vi "AlGaInPAs_run_dil_v11.vi"(2 "Debug Mode":bool, 3 "Elapsed Time(s)":dbl, 4 "State":enum16{"Edit", "Start", "Run", "End", "Idle"}(ring), 5 "Argument List In":string[](array[string])) -> (0 "Status Out":string, 1 "Argument List Out":string[](array[string]))   [LabVIEW 2011]
panel:
  out "Prep-Ga var":bool
  out "run started":bool
  out "first":bool=TRUE
  out "total time":dbl
  out "is OK?":bool
  out "AsH3?":bool
  out "PH3?":bool
  out "In?":bool
  out "Ga?":bool
  out "Al?":bool
  in  "Run As":bool caption="Run"
  in  "AsH3 Flow":dbl caption="AsH3 Flow (0-10 sccm)" format="%.2f"
  in  "P Flow":dbl caption="P Flow (0-100 sccm)" format="%.2f"
  in  "Run P":bool caption="Run"
  in  "In Flow":dbl caption="In Flow (0-100 sscm)" format="%.2f"
  in  "Run In":bool caption="Run"
  in  "Run Al":bool caption="Run"
  in  "Al Flow":dbl caption="Al Flow (0-100 sscm)" format="%.2f"
  in  "Cancel":bool
  in  "OK":bool
  out "tTotal(s) 2":dbl
  in  "Ga Tab Control":enum32{"Page 1", "Page 2"}(tab)
  in  "Ga Dilution":bool caption="Dilute"
  in  "Ga Flow":dbl caption="Ga Flow (0-10 sscm)" format="%.2f"
  in  "Run Ga":bool caption="Run"
  in  "GAMFC1":dbl=1.0 caption="R1 (0-10 sscm)" format="%.2f"
  out "GAMFC2 set":dbl caption="R2 (0-100 sscm)" format="%.2f"
  in  "GAMFC3":dbl=100.0 caption="R3 (0-1000 sscm)" format="%.1f"
  out "GAMFC1 set":dbl caption="R1 (0-10 sscm)" format="%.2f"
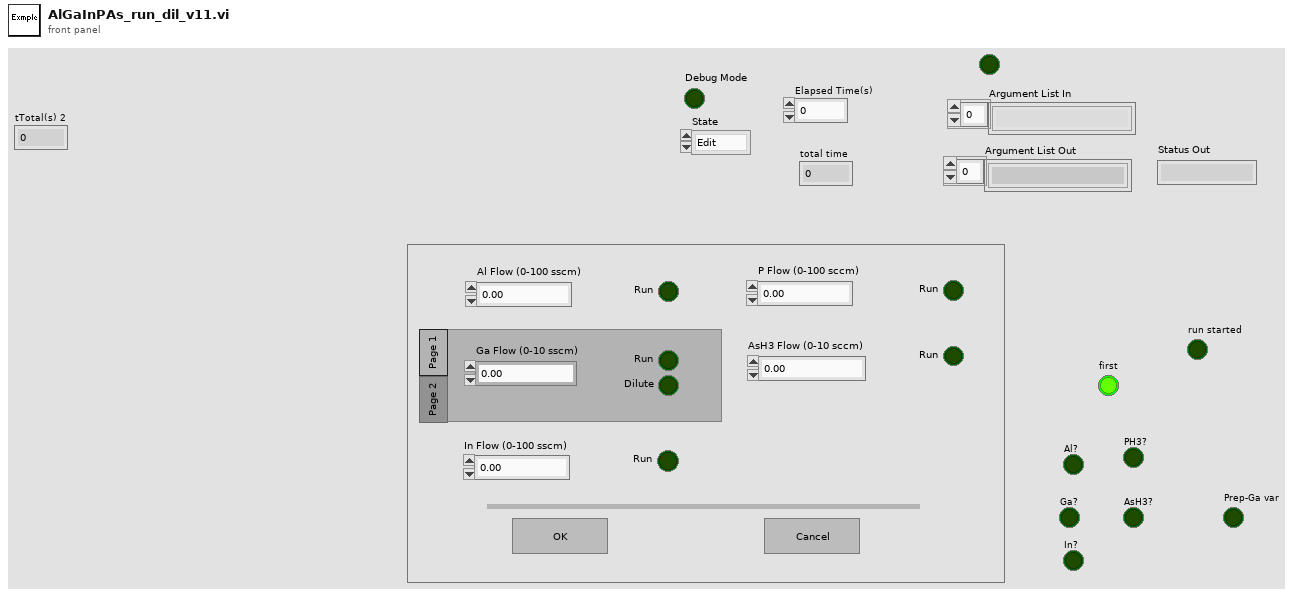
[diagram p1: front panel]
types:
  T1 = enum16{"Discrete", "Continuous", "Instantaneous", "Finite"}
  T2 = enum32{"Invalid", "Default", "Floating", "Floating/Auto-Hide", "Modal"}
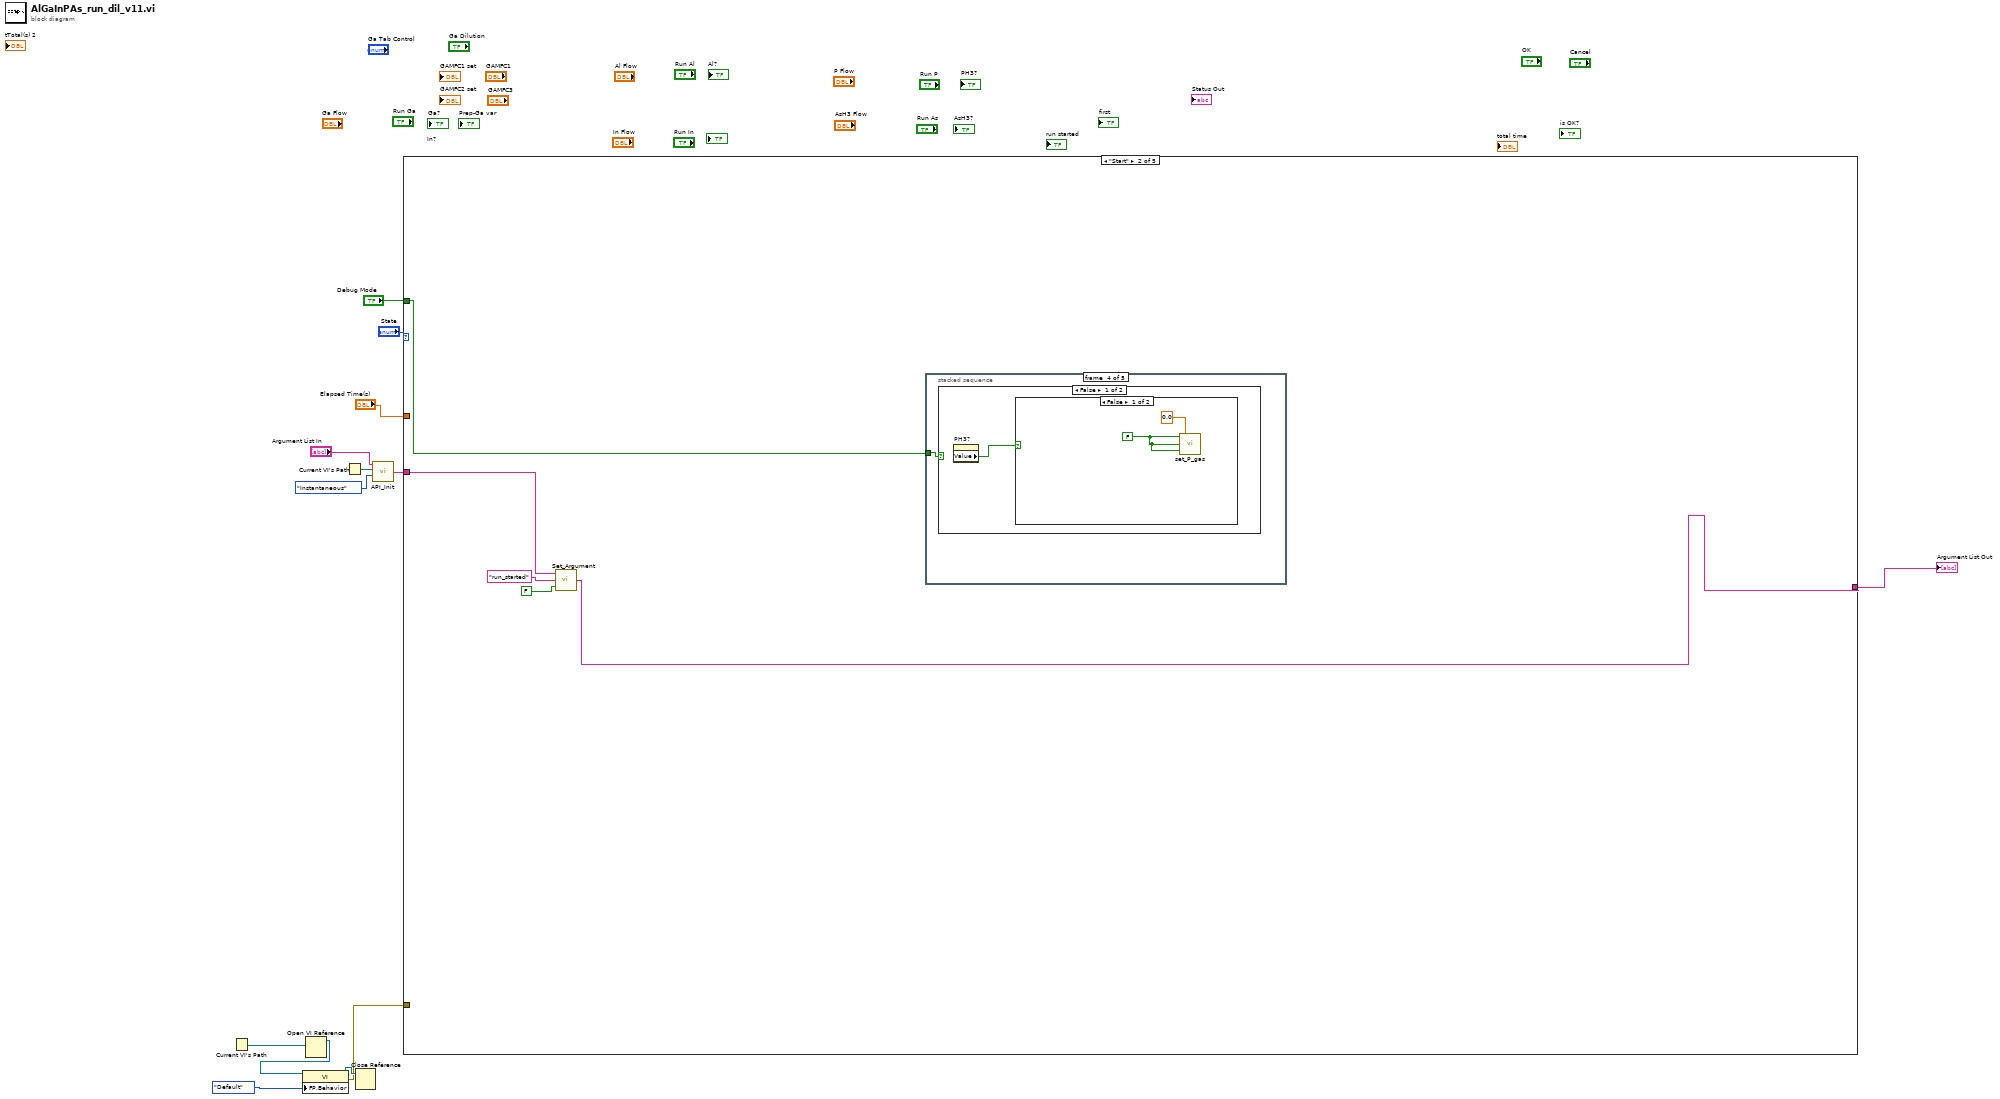
[diagram p0: block diagram]
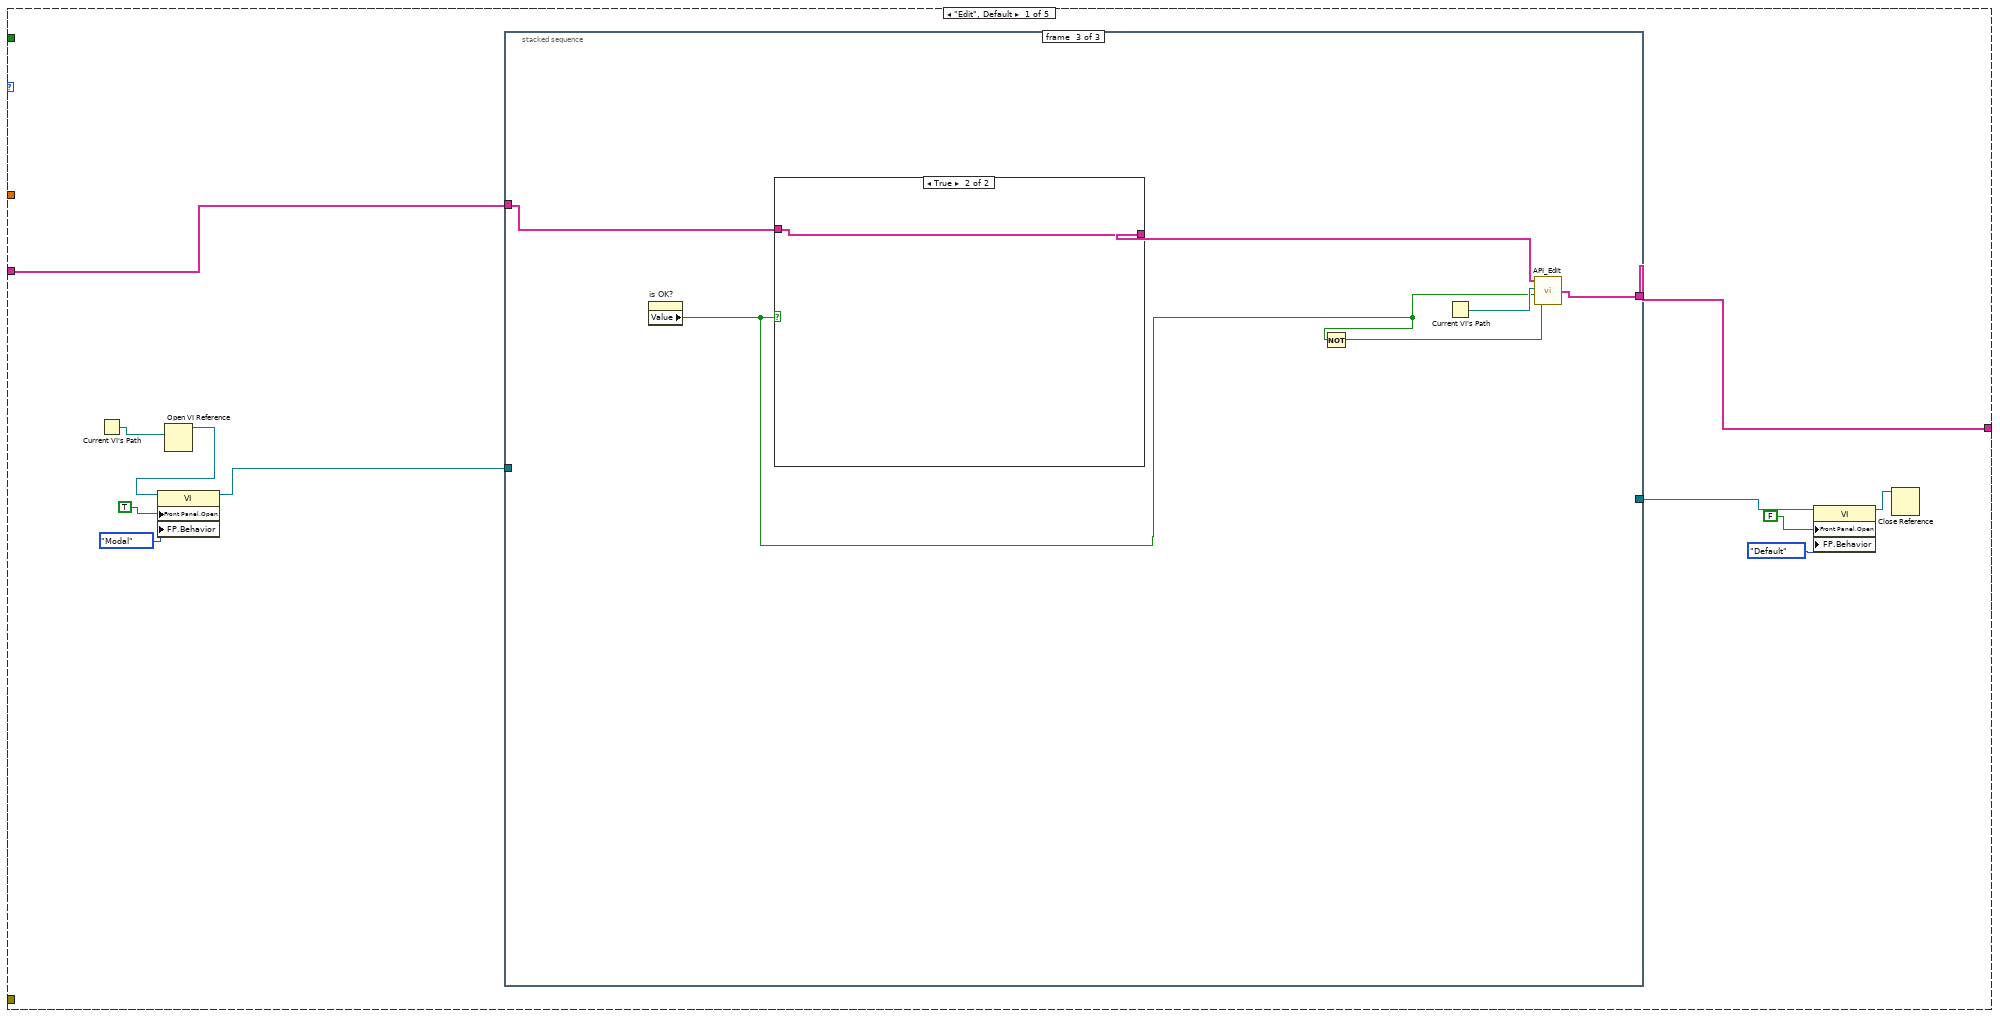
[diagram p2: hidden frame]
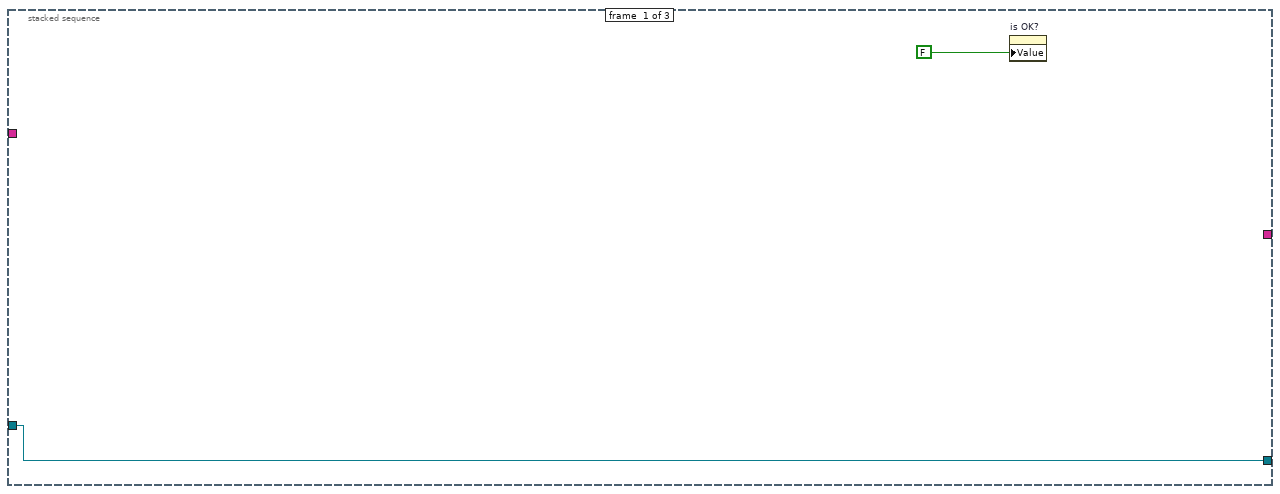
[diagram p3: hidden frame]
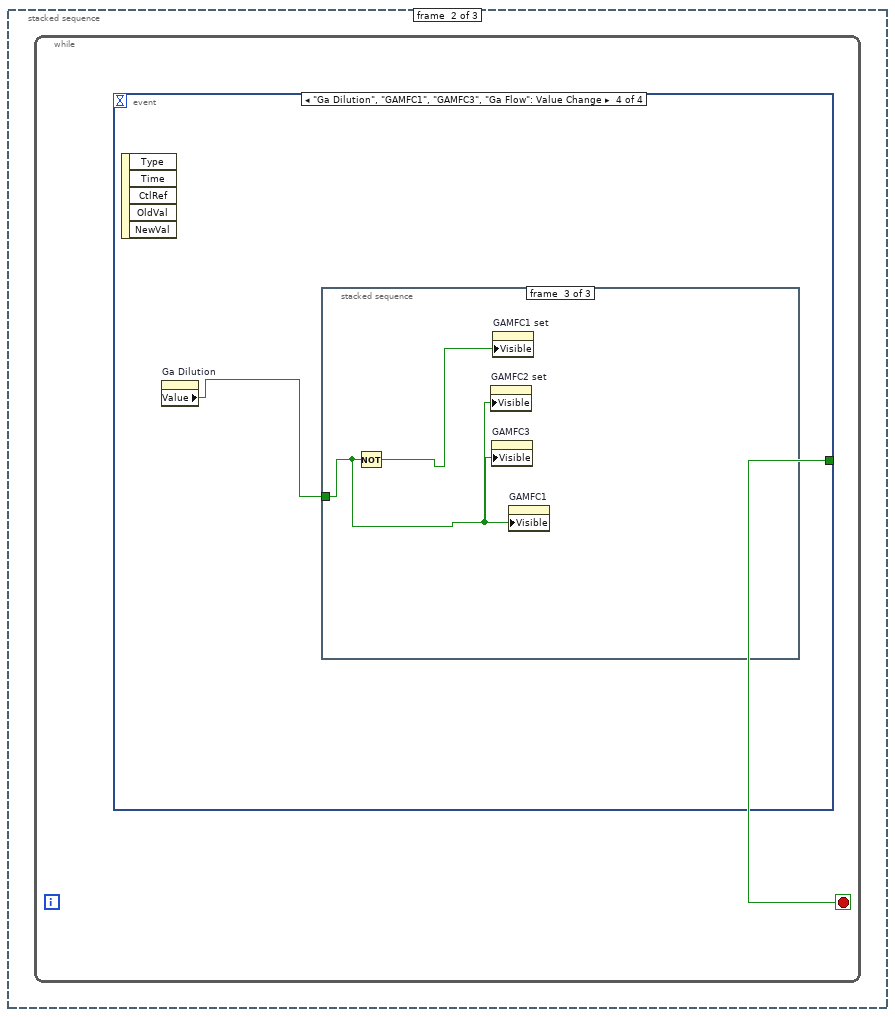
[diagram p4: hidden frame]
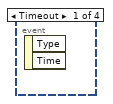
[diagram p5: hidden frame]
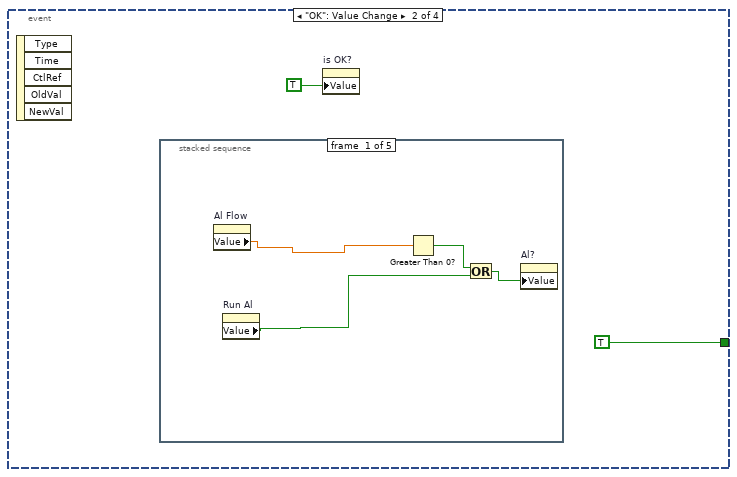
[diagram p6: hidden frame]
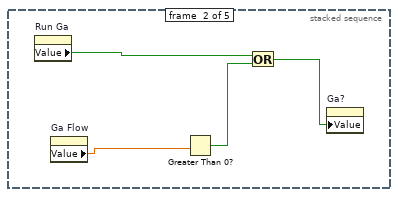
[diagram p7: hidden frame]
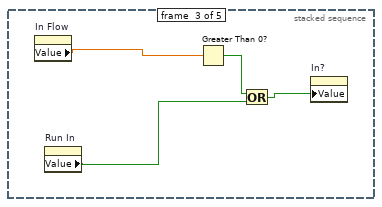
[diagram p8: hidden frame]
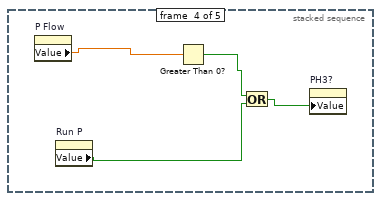
[diagram p9: hidden frame]
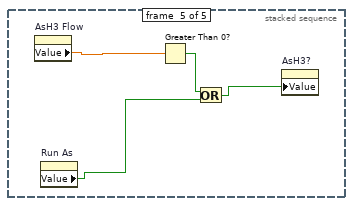
[diagram p10: hidden frame]
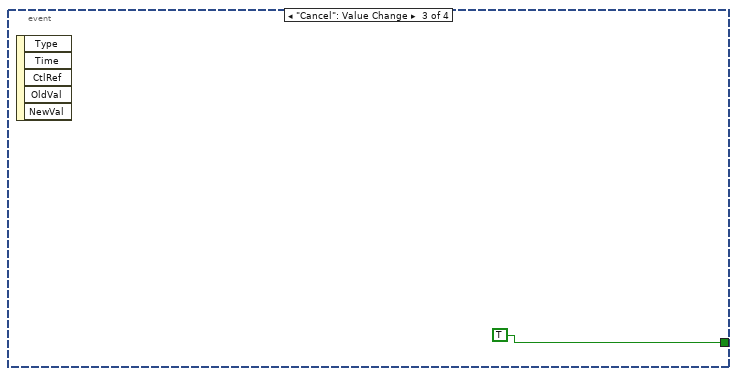
[diagram p11: hidden frame]
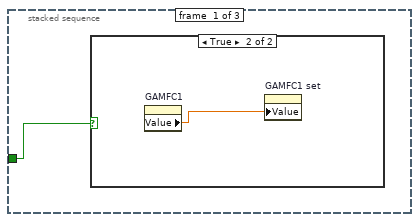
[diagram p12: hidden frame]
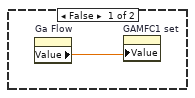
[diagram p13: hidden frame]
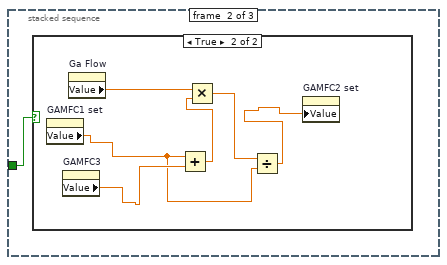
[diagram p14: hidden frame]
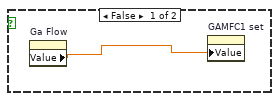
[diagram p15: hidden frame]
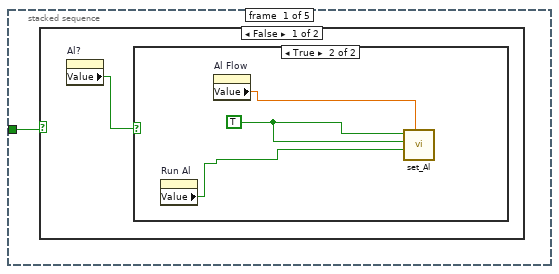
[diagram p17: hidden frame]
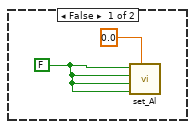
[diagram p18: hidden frame]
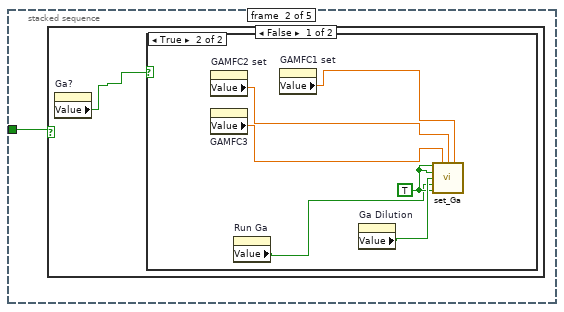
[diagram p20: hidden frame]
diagram:
  n1 = Current VI's Path() -> (path=w9:path)
  n2 = Open VI Reference(vi path=w9) -> (vi reference=w8:refnum<vi>)  [unwired: 1 in, 5 out]
  n3 = property class="VI"(reference=w8, "FP.Behavior"=T2."Default" ("Front Panel Window:Behavior")) -> (reference out=w6:refnum<vi>, error out=w5:errorcluster)  [unwired: 1 in]
  n4 = Current VI's Path() -> (path=w4:path)
  n5 = Close Reference(reference=w6) -> ()  [unwired: 1 in, 1 out]
  n6 = call "API_Init.vi"("API Mode"=T1."Instantaneous", "VI Path"=w4, "Argument List In"="Argument List In") -> ("Argument List Out"=w1:string[])  [unwired: 1 in]
  n7 = case shown="\"Start\"" "State" {
    tunnel: "Debug Mode" -> [_ w73 w117 _ _]
    tunnel: "Elapsed Time(s)" -> [_ _ w119 _ _]
    tunnel: w1 -> [w15 w75 w116 w162 w163]
    tunnel: [w14 w74 w118 w162 w163] -> w10
    tunnel: w5 -> [_ _ _ _ _]
    frame "Edit", Default {
      n8 = Current VI's Path() -> (path=w20:path)
      n9 = Open VI Reference(vi path=w20) -> (vi reference=w19:refnum<vi>)  [unwired: 1 in, 5 out]
      n10 = property class="VI"(reference=w19, "Front Panel.Open"=TRUE ("Front Panel Window:Open"), "FP.Behavior"=T2."Modal" ("Front Panel Window:Behavior")) -> (reference out=w18:refnum<vi>)  [unwired: 1 in, 1 out]
      n11 = stacked-sequence {
        tunnel: w15 -> [_ _ w68]
        tunnel: w18 -> [w26 _ _]
        tunnel: [w26 _ _] -> w22
        tunnel: [_ _ w66] -> w14
        frame #0 {
          n12 = property on="is OK?" class="Bool (strict)"("Value"=FALSE ("is OK?")) -> ()  [unwired: 2 in, 2 out]
        }
        frame #1 {
          n13 = while {
            stop <- w27 stop-if-true
            n14 = event shown="[3] \"Ga Dilution\", \"GAMFC1\", \"GAMFC3\", \"Ga Flow\": Value Change" {
              selector: _ -> [_ _ _ _]
              dyn-events: _ -> [_ _ _ _]
              timeout: _ -> [_ _ _ _]
              tunnel: [_ TRUE TRUE _] -> w27
              event Timeout {
                n15 = event-data() -> ()  [unwired: 1 in, 2 out]
              }
              event "OK": Value Change {
                n16 = event-data() -> ()  [unwired: 1 in, 5 out]
                n17 = stacked-sequence {
                  frame #0 {
                    n18 = property on="Al Flow" class="DigNum (strict)"() -> ("Value"=w32:dbl)  [unwired: 2 in, 2 out]
                    n19 = property on="Run Al" class="Bool (strict)"() -> ("Value"=w31:bool)  [unwired: 2 in, 2 out]
                    n20 = Greater Than 0?(x=w32) -> (x > 0?=w33:bool)
                    n21 = Or(x=w33, y=w31) -> (x .or. y?=w30:bool)
                    n22 = property on="Al?" class="Bool (strict)"("Value"=w30) -> ()  [unwired: 2 in, 2 out]
                  }
                  frame #1 {
                    n23 = property on="Run Ga" class="Bool (strict)"() -> ("Value"=w35:bool)  [unwired: 2 in, 2 out]
                    n24 = property on="Ga Flow" class="DigNum (strict)"() -> ("Value"=w36:dbl)  [unwired: 2 in, 2 out]
                    n25 = Greater Than 0?(x=w36) -> (x > 0?=w37:bool)
                    n26 = Or(x=w35, y=w37) -> (x .or. y?=w34:bool)
                    n27 = property on="Ga?" class="Bool (strict)"("Value"=w34) -> ()  [unwired: 2 in, 2 out]
                  }
                  frame #2 {
                    n28 = property on="In Flow" class="DigNum (strict)"() -> ("Value"=w39:dbl)  [unwired: 2 in, 2 out]
                    n29 = property on="Run In" class="Bool (strict)"() -> ("Value"=w40:bool)  [unwired: 2 in, 2 out]
                    n30 = Greater Than 0?(x=w39) -> (x > 0?=w41:bool)
                    n31 = Or(x=w41, y=w40) -> (x .or. y?=w38:bool)
                    n32 = property on="In?" class="Bool (strict)"("Value"=w38) -> ()  [unwired: 2 in, 2 out]
                  }
                  frame #3 {
                    n33 = property on="P Flow" class="DigNum (strict)"() -> ("Value"=w44:dbl)  [unwired: 2 in, 2 out]
                    n34 = property on="Run P" class="Bool (strict)"() -> ("Value"=w43:bool)  [unwired: 2 in, 2 out]
                    n35 = Greater Than 0?(x=w44) -> (x > 0?=w45:bool)
                    n36 = Or(x=w45, y=w43) -> (x .or. y?=w42:bool)
                    n37 = property on="PH3?" class="Bool (strict)"("Value"=w42) -> ()  [unwired: 2 in, 2 out]
                  }
                  frame #4 {
                    n38 = property on="AsH3 Flow" class="DigNum (strict)"() -> ("Value"=w48:dbl)  [unwired: 2 in, 2 out]
                    n39 = property on="Run As" class="Bool (strict)"() -> ("Value"=w47:bool)  [unwired: 2 in, 2 out]
                    n40 = Greater Than 0?(x=w48) -> (x > 0?=w49:bool)
                    n41 = Or(x=w49, y=w47) -> (x .or. y?=w46:bool)
                    n42 = property on="AsH3?" class="Bool (strict)"("Value"=w46) -> ()  [unwired: 2 in, 2 out]
                  }
                }
                n43 = property on="is OK?" class="Bool (strict)"("Value"=TRUE ("is OK?")) -> ()  [unwired: 2 in, 2 out]
              }
              event "Cancel": Value Change {
                n44 = event-data() -> ()  [unwired: 1 in, 5 out]
              }
              event "Ga Dilution", "GAMFC1", "GAMFC3", "Ga Flow": Value Change {
                n45 = event-data() -> ()  [unwired: 1 in, 5 out]
                n46 = property on="Ga Dilution" class="Bool (strict)"() -> ("Value"=w51:bool)  [unwired: 2 in, 2 out]
                n47 = stacked-sequence {
                  tunnel: w51 -> [w52 w55 w63]
                  frame #0 {
                    n48 = case shown="True" w52 {
                      frame False {
                        n49 = property on="Ga Flow" class="DigNum (strict)"() -> ("Value"=w53:dbl)  [unwired: 2 in, 2 out]
                        n50 = property on="GAMFC1 set" class="DigNum (strict)"("Value"=w53) -> ()  [unwired: 2 in, 2 out]
                      }
                      frame True {
                        n51 = property on="GAMFC1" class="DigNum (strict)"() -> ("Value"=w54:dbl)  [unwired: 2 in, 2 out]
                        n52 = property on="GAMFC1 set" class="DigNum (strict)"("Value"=w54) -> ()  [unwired: 2 in, 2 out]
                      }
                    }
                  }
                  frame #1 {
                    n53 = case shown="True" w55 {
                      frame False {
                        n54 = property on="Ga Flow" class="DigNum (strict)"() -> ("Value"=w56:dbl)  [unwired: 2 in, 2 out]
                        n55 = property on="GAMFC1 set" class="DigNum (strict)"("Value"=w56) -> ()  [unwired: 2 in, 2 out]
                      }
                      frame True {
                        n56 = property on="GAMFC1 set" class="DigNum (strict)"() -> ("Value"=w57:dbl)  [unwired: 2 in, 2 out]
                        n57 = property on="GAMFC3" class="DigNum (strict)"() -> ("Value"=w59:dbl)  [unwired: 2 in, 2 out]
                        n58 = property on="Ga Flow" class="DigNum (strict)"() -> ("Value"=w60:dbl)  [unwired: 2 in, 2 out]
                        n59 = Add(x=w57, y=w59) -> (x+y=w62:dbl)
                        n60 = Multiply(x=w60, y=w62) -> (x*y=w58:dbl)
                        n61 = Divide(x=w58, y=w57) -> (x/y=w61:dbl)
                        n62 = property on="GAMFC2 set" class="DigNum (strict)"("Value"=w61) -> ()  [unwired: 2 in, 2 out]
                      }
                    }
                  }
                  frame #2 {
                    n63 = Not(x=w63) -> (.not. x?=w64:bool)
                    n64 = property on="GAMFC2 set" class="DigNum (strict)"("Visible"=w63) -> ()  [unwired: 2 in, 2 out]
                    n65 = property on="GAMFC3" class="DigNum (strict)"("Visible"=w63) -> ()  [unwired: 2 in, 2 out]
                    n66 = property on="GAMFC1 set" class="DigNum (strict)"("Visible"=w64) -> ()  [unwired: 2 in, 2 out]
                    n67 = property on="GAMFC1" class="DigNum (strict)"("Visible"=w63) -> ()  [unwired: 2 in, 2 out]
                  }
                }
              }
            }
          }
        }
        frame #2 {
          n68 = property on="is OK?" class="Bool (strict)"() -> ("Value"=w65:bool)  [unwired: 2 in, 2 out]
          n69 = case shown="True" w65 {
            tunnel: w68 -> [w71 w72]
            tunnel: [w71 w72] -> w67
            frame False {
            }
            frame True {
            }
          }
          n70 = Not(x=w65) -> (.not. x?=w70:bool)
          n71 = Current VI's Path() -> (path=w69:path)
          n72 = call "API_Edit.vi"("Cancel"=w70, "OK"=w65, "VI Path"=w69, "Argument List In"=w67) -> ("Argument List Out"=w66:string[])
        }
      }
      n73 = property class="VI"(reference=w22, "Front Panel.Open"=FALSE ("Front Panel Window:Open"), "FP.Behavior"=T2."Default" ("Front Panel Window:Behavior")) -> (reference out=w23:refnum<vi>)  [unwired: 1 in, 1 out]
      n74 = Close Reference(reference=w23) -> ()  [unwired: 1 in, 1 out]
    }
    frame "Start" {
      n75 = call "Set_Argument.vi"("Enable"=FALSE, "Argument"="run_started", "Argument List In"=w75) -> ("Argument List Out"=w74:string[])
      n76 = stacked-sequence {
        tunnel: w73 -> [w78 w85 w95 w102 w109]
        frame #0 {
          n77 = case shown="False" w78 {
            frame False {
              n78 = property on="Al?" class="Bool (strict)"() -> ("Value"=w79:bool)  [unwired: 2 in, 2 out]
              n79 = case shown="True" w79 {
                frame False {
                  w80 = FALSE ("Al Active")
                  n80 = call "set_Al.vi"("ALMFC1"=0.0 ("Aluminum Flow"), "Remote"=w80, "Run"=w80, "Bubbler In"=w80, "Active"=w80) -> ()  [unwired: 5 out]
                }
                frame True {
                  w84 = TRUE ("Al Active")
                  n81 = property on="Run Al" class="Bool (strict)"() -> ("Value"=w82:bool)  [unwired: 2 in, 2 out]
                  n82 = property on="Al Flow" class="DigNum (strict)"() -> ("Value"=w83:dbl)  [unwired: 2 in, 2 out]
                  n83 = call "set_Al.vi"("ALMFC1"=w83, "Run"=w82, "Bubbler In"=w84, "Active"=w84) -> ()  [unwired: 1 in, 5 out]
                }
              }
            }
            frame True {
            }
          }
        }
        frame #1 {
          n84 = case shown="False" w85 {
            frame False {
              n85 = property on="Ga?" class="Bool (strict)"() -> ("Value"=w86:bool)  [unwired: 2 in, 2 out]
              n86 = case shown="True" w86 {
                frame False {
                  w88 = FALSE ("Ga Active")
                  w87 = 0.0 ("Ga Flow 1")
                  n87 = call "set_Ga.vi"("Active"=w88, "GAMFC3"=w87, "GAMFC2"=w87, "GAMFC1"=w87, "Bubbler In"=w88, "H2 Dilute"=w88, "Run"=w88, "Remote"=w88) -> ()  [unwired: 8 out]
                }
                frame True {
                  w90 = TRUE ("Ga Active")
                  n88 = property on="GAMFC2 set" class="DigNum (strict)"() -> ("Value"=w92:dbl)  [unwired: 2 in, 2 out]
                  n89 = property on="GAMFC3" class="DigNum (strict)"() -> ("Value"=w91:dbl)  [unwired: 2 in, 2 out]
                  n90 = property on="Run Ga" class="Bool (strict)"() -> ("Value"=w89:bool)  [unwired: 2 in, 2 out]
                  n91 = property on="GAMFC1 set" class="DigNum (strict)"() -> ("Value"=w93:dbl)  [unwired: 2 in, 2 out]
                  n92 = property on="Ga Dilution" class="Bool (strict)"() -> ("Value"=w94:bool)  [unwired: 2 in, 2 out]
                  n93 = call "set_Ga.vi"("Active"=w90, "GAMFC3"=w91, "GAMFC2"=w92, "GAMFC1"=w93, "Bubbler In"=w90, "H2 Dilute"=w94, "Run"=w89, "Remote"=w90) -> ()  [unwired: 8 in]
                }
              }
            }
            frame True {
            }
          }
        }
        frame #2 {
          n94 = case shown="False" w95 {
            frame False {
              n95 = property on="In?" class="Bool (strict)"() -> ("Value"=w96:bool)  [unwired: 2 in, 2 out]
              n96 = case shown="True" w96 {
                frame False {
                  w98 = FALSE ("In Remote")
                  n97 = call "set_In.vi"("INMFC1"=0.0 ("Indium Flow"), "Remote"=w98, "Run"=w98, "Bubbler In"=w98, "Active"=w98) -> ()  [unwired: 5 out]
                }
                frame True {
                  w101 = TRUE ("In Run")
                  n98 = property on="Run In" class="Bool (strict)"() -> ("Value"=w99:bool)  [unwired: 2 in, 2 out]
                  n99 = property on="In Flow" class="DigNum (strict)"() -> ("Value"=w100:dbl)  [unwired: 2 in, 2 out]
                  n100 = call "set_In.vi"("INMFC1"=w100, "Run"=w99, "Bubbler In"=w101, "Active"=w101) -> ()  [unwired: 1 in, 5 out]
                }
              }
            }
            frame True {
            }
          }
        }
        frame #3 {
          n101 = case shown="False" w102 {
            frame False {
              n102 = property on="PH3?" class="Bool (strict)"() -> ("Value"=w103:bool)  [unwired: 2 in, 2 out]
              n103 = case shown="False" w103 {
                frame False {
                  w104 = FALSE ("P_Gas Active")
                  n104 = call "set_P_gas.vi"("Run"=w104, "Gas In"=w104, "Active"=w104, "P_Gas Remote"=w104, "H2 Flush"=w104, "P_Gas Flow"=0.0) -> ()
                }
                frame True {
                  w108 = TRUE ("P_Gas Active")
                  n105 = property on="P Flow" class="DigNum (strict)"() -> ("Value"=w107:dbl)  [unwired: 2 in, 2 out]
                  n106 = property on="Run P" class="Bool (strict)"() -> ("Value"=w106:bool)  [unwired: 2 in, 2 out]
                  n107 = call "set_P_gas.vi"("Active"=w108, "P_Gas Remote"=w106, "H2 Flush"=w108, "P_Gas Flow"=w107) -> ()  [unwired: 2 in]
                }
              }
            }
            frame True {
            }
          }
        }
        frame #4 {
          n108 = case shown="False" w109 {
            frame False {
              n109 = property on="AsH3?" class="Bool (strict)"() -> ("Value"=w110:bool)  [unwired: 2 in, 2 out]
              n110 = case shown="True" w110 {
                frame False {
                  w111 = FALSE ("As_Gas Active")
                  n111 = call "set_As_gas.vi"("Active"=w111, "As_Gas Flow"=0.0, "Gas In"=w111, "H2 Flush"=w111, "Run"=w111, "Remote"=w111) -> ()  [unwired: 10 in]
                }
                frame True {
                  w115 = TRUE ("As_Gas Active")
                  n112 = property on="Run As" class="Bool (strict)"() -> ("Value"=w113:bool)  [unwired: 2 in, 2 out]
                  n113 = property on="AsH3 Flow" class="DigNum (strict)"() -> ("Value"=w114:dbl)  [unwired: 2 in, 2 out]
                  n114 = call "set_As_gas.vi"("Active"=w115, "As_Gas Flow"=w114, "Gas In"=w115, "Run"=w113) -> ()  [unwired: 12 in]
                }
              }
            }
            frame True {
            }
          }
        }
      }
    }
    frame "Run" {
      n115 = stacked-sequence {
        tunnel: w119 -> [_ _]
        tunnel: w116 -> [_ w161]
        tunnel: [_ w161] -> w118
        tunnel: w117 -> [_ _]
        frame #0 {
          n116 = stacked-sequence {
            frame #0 {
              n117 = property on="Status Out" class="Str"("Value"="run: ") -> ()  [unwired: 2 in, 2 out]
            }
            frame #1 {
              w121 = FALSE ("prep source?")
              n118 = property on="Status Out" class="Str"() -> ("Value"=w127:string)  [unwired: 2 in, 2 out]
              n119 = property on="Al?" class="Bool (strict)"() -> ("Value"=w128:bool)  [unwired: 2 in, 2 out]
              n120 = property on="Run Al" class="Bool (strict)"() -> ("Value"=w122:bool)  [unwired: 2 in, 2 out]
              n121 = call "flow_strings.vi"("string in"=w127, "is first in?"=TRUE, "use source?"=w128, "name"="Al", "run source?"=w122, "prep source?"=w121, "is prep?"=w121) -> ("string out"=w126:string, "is first out?"=w125:bool)
              n122 = property on="Status Out" class="Str"("Value"=w126) -> ()  [unwired: 2 in, 2 out]
              n123 = property on="first" class="Bool (strict)"("Value"=w125) -> ()  [unwired: 2 in, 2 out]
            }
            frame #2 {
              w129 = FALSE ("prep source?")
              n124 = property on="first" class="Bool (strict)"() -> ("Value"=w132:bool)  [unwired: 2 in, 2 out]
              n125 = property on="Status Out" class="Str"() -> ("Value"=w135:string)  [unwired: 2 in, 2 out]
              n126 = property on="Ga?" class="Bool (strict)"() -> ("Value"=w133:bool)  [unwired: 2 in, 2 out]
              n127 = property on="Run Ga" class="Bool (strict)"() -> ("Value"=w130:bool)  [unwired: 2 in, 2 out]
              n128 = call "flow_strings.vi"("string in"=w135, "is first in?"=w132, "use source?"=w133, "name"="Ga", "run source?"=w130, "prep source?"=w129, "is prep?"=w129) -> ("string out"=w136:string, "is first out?"=w131:bool)
              n129 = property on="Status Out" class="Str"("Value"=w136) -> ()  [unwired: 2 in, 2 out]
              n130 = property on="first" class="Bool (strict)"("Value"=w131) -> ()  [unwired: 2 in, 2 out]
            }
            frame #3 {
              w137 = FALSE ("is prep?")
              n131 = property on="first" class="Bool (strict)"() -> ("Value"=w141:bool)  [unwired: 2 in, 2 out]
              n132 = property on="Status Out" class="Str"() -> ("Value"=w143:string)  [unwired: 2 in, 2 out]
              n133 = property on="In?" class="Bool (strict)"() -> ("Value"=w144:bool)  [unwired: 2 in, 2 out]
              n134 = property on="Run In" class="Bool (strict)"() -> ("Value"=w138:bool)  [unwired: 2 in, 2 out]
              n135 = call "flow_strings.vi"("string in"=w143, "is first in?"=w141, "use source?"=w144, "name"="In", "run source?"=w138, "prep source?"=w137, "is prep?"=w137) -> ("string out"=w140:string, "is first out?"=w139:bool)
              n136 = property on="Status Out" class="Str"("Value"=w140) -> ()  [unwired: 2 in, 2 out]
              n137 = property on="first" class="Bool (strict)"("Value"=w139) -> ()  [unwired: 2 in, 2 out]
            }
            frame #4 {
              w145 = FALSE ("prep source?")
              n138 = property on="first" class="Bool (strict)"() -> ("Value"=w148:bool)  [unwired: 2 in, 2 out]
              n139 = property on="Status Out" class="Str"() -> ("Value"=w150:string)  [unwired: 2 in, 2 out]
              n140 = property on="PH3?" class="Bool (strict)"() -> ("Value"=w151:bool)  [unwired: 2 in, 2 out]
              n141 = property on="Run P" class="Bool (strict)"() -> ("Value"=w146:bool)  [unwired: 2 in, 2 out]
              n142 = call "flow_strings.vi"("string in"=w150, "is first in?"=w148, "use source?"=w151, "name"="P", "run source?"=w146, "prep source?"=w145, "is prep?"=w145) -> ("string out"=w149:string, "is first out?"=w147:bool)
              n143 = property on="Status Out" class="Str"("Value"=w149) -> ()  [unwired: 2 in, 2 out]
              n144 = property on="first" class="Bool (strict)"("Value"=w147) -> ()  [unwired: 2 in, 2 out]
            }
            frame #5 {
              w153 = FALSE ("prep source?")
              n145 = property on="first" class="Bool (strict)"() -> ("Value"=w156:bool)  [unwired: 2 in, 2 out]
              n146 = property on="Status Out" class="Str"() -> ("Value"=w158:string)  [unwired: 2 in, 2 out]
              n147 = property on="AsH3?" class="Bool (strict)"() -> ("Value"=w159:bool)  [unwired: 2 in, 2 out]
              n148 = property on="Run As" class="Bool (strict)"() -> ("Value"=w154:bool)  [unwired: 2 in, 2 out]
              n149 = call "flow_strings.vi"("string in"=w158, "is first in?"=w156, "use source?"=w159, "name"="As", "run source?"=w154, "prep source?"=w153, "is prep?"=w153) -> ("string out"=w155:string, "is first out?"=w157:bool)
              n150 = property on="Status Out" class="Str"("Value"=w155) -> ()  [unwired: 2 in, 2 out]
              n151 = property on="first" class="Bool (strict)"("Value"=w157) -> ()  [unwired: 2 in, 2 out]
            }
          }
        }
        frame #1 {
        }
      }
    }
    frame "End" {
    }
    frame "Idle" {
    }
  }
  "Argument List Out" <- w10
